vi "Remove CEID.vi"(8 "error in (no error)":errorcluster, 11 "CEID":u32[](array[numeric])) -> (0 "error out":errorcluster)   [LabVIEW 2020, in "SECS Communication.lvlib" / "SECS Data Class.lvclass"]
uses:
  SECS Data Class.lvclass
  SECS Data Class.lvclass/SECS Data Class.ctl
  Get All CEID Data.vi
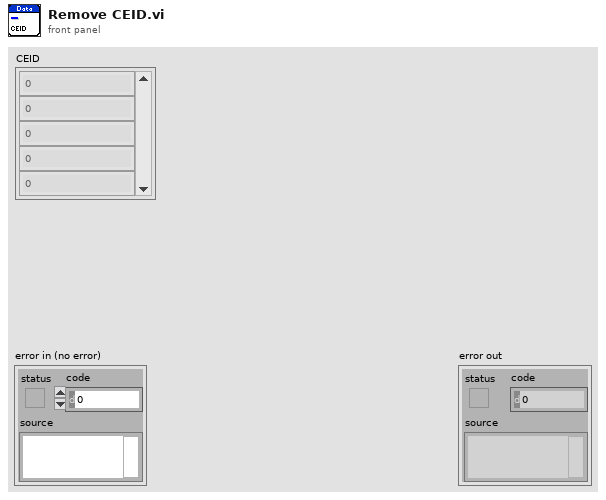
[diagram p1: front panel]
types:
  T1 = typedef "SECS Communication.lvlib/SECS Data Class.lvclass/CEID Data.ctl" = cluster{"Enable":bool, "CEID":u32, "Name":string, "Description":string, "RPTID":u32[], "Dynamic":bool}
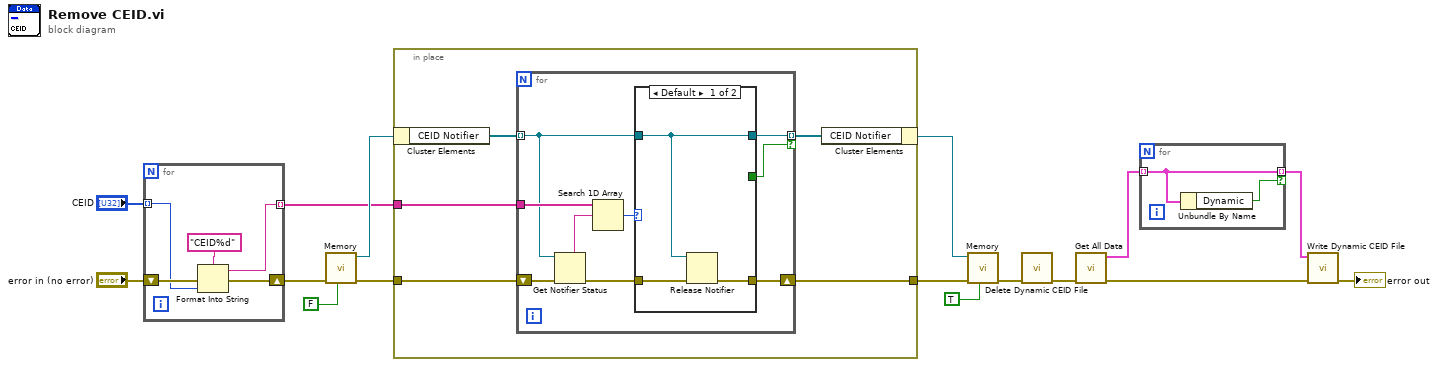
[diagram p0: block diagram]
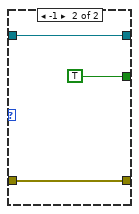
[diagram p2: hidden frame]
diagram:
  n1 = for {
    shift-right: [w19] -> w10
    shift-left: "error in (no error)" -> [w21]
    tunnel: "CEID" -> [w18] mode=indexing
    tunnel: [w17] -> w8 mode=indexing
    n2 = Format Into String(format string="CEID%d", error in=w21, w18) -> (resulting string=w17:string, error out=w19:errorcluster)  [unwired: 1 in]
  }
  n3 = call "Memory.vi"("Put"=FALSE, "error in (no error)"=w10) -> ("error out"=w14:errorcluster, "SECS Data Class out"=w15:refnum<class "SECS Data Class.lvclass">)  [unwired: 8 in]
  n4 = in-place {
    in-place-border: w14 -> [w26]
    in-place-border: w8 -> [w25]
    in-place-border: [w22] -> w7
    n5 = in-place-cluster #1(w15) -> ("CEID Notifier"=w24:refnum<notifier>[])
    n6 = for {
      tunnel: w25 -> [w34]
      tunnel: w24 -> [w31] mode=indexing
      tunnel: [w30] -> w23 mode=indexing if=w27
      shift-right: [w28] -> w22
      shift-left: w26 -> [w35]
      n7 = Get Notifier Status(notifier=w31, error in (no error)=w35) -> (notifier name=w33:string, error out=w29:errorcluster)  [unwired: 3 out]
      n8 = Search 1D Array(1D array=w34, element=w33) -> (index of element=w32:i32)  [unwired: 1 in]
      n9 = case shown="Default" w32 {
        tunnel: w31 -> [w37 w41]
        tunnel: [w37 w41] -> w30
        tunnel: w29 -> [w38 w40]
        tunnel: [w36 w40] -> w28
        tunnel: [_ TRUE] -> w27
        frame Default {
          n10 = Release Notifier(notifier=w37, error in (no error)=w38) -> (error out=w36:errorcluster)  [unwired: 1 in, 2 out]
        }
        frame -1 {
        }
      }
    }
    n11 = in-place-cluster #1("CEID Notifier"=w23) -> (w13:refnum<class "SECS Data Class.lvclass">)
  }
  n12 = call "Memory.vi"("Put"=TRUE, "error in (no error)"=w7, "SECS Data Class in"=w13) -> ("error out"=w5:errorcluster)  [unwired: 7 in, 1 out]
  n13 = call "Delete Dynamic CEID File.vi"("error in (no error)"=w5) -> ("error out"=w4:errorcluster)  [unwired: 10 in]
  n14 = call-poly "Get All Data.vi"("error in (no error)"=w4) -> ("error out"=w3:errorcluster, "CEID Data"=w6:T1[])  [unwired: 9 in]
  n15 = for {
    tunnel: w6 -> [w43] mode=indexing
    tunnel: [w43] -> w2 mode=indexing if=w42
    n16 = Unbundle By Name(w43) -> ("Dynamic"=w42:bool)
  }
  n17 = call "Write Dynamic CEID File.vi"("error in (no error)"=w3, "CEID Data In"=w2) -> ("error out"=→"error out":errorcluster)  [unwired: 9 in]
